vi "driverdata.vi"() -> ()   [LabVIEW 2020]
doc: "This global variable contains data from the FMS system as well as the FRC 4265 Dashboard including safety overrides, calibration commands, and configuration parameters. These data are updated during all robot modes. Robot commands should never be placed in this global variable."
uses:
  <vilib>/Rock Robotics/WPI/DriverStation/WPI_DriverStationRobotMode2.ctl
  <vilib>/Rock Robotics/WPI/DriverStation/WPI_DriverStationAllianceInfo.ctl
panel:
  out "TCP_Override":bool
  out "Starting_TCP_Override":bool
  out "Some_Switch_Armed":bool
  out "Free_Tuning_Variable":dbl
  out "Apply_HUB_Height_Offset":bool
  out "Remaining_Time":dbl
  out "Alliance_Color":T1
  out "Dashboard_Tab":i8
  out "Running_Systems_Check":bool
  out "New_Driver_Profile_Setpoints":dbl[](array[numeric])
  out "Apply_Driver_Profile_Setpoints":bool
  out "Starting_Safety_Override":bool
  out "Starting_IMU_Reset":bool
  out "Field_Oriented_Override":bool
  out "Driver_DPad":T2(ring)
  out "Force_Human_Control":bool
  out "Test_Actuator_Period (s)":dbl
  out "Driver_Joystick_Calibrations":dbl[](array[numeric])
  out "Robot_is_Autonomous":bool
  out "Test_Actuator_Value":dbl
  out "Test_Actuator_Name":string
  out "Disable_Fusion_While_Autonomous":bool
  out "Disable_Fusion_While_Disabled":bool
  out "Camera_Override":bool
  out "Auto_Test_Mode":bool
  out "Clear_Errors":bool
  out "Master_Safety_Override":bool
  out "Auto_Delay (s)":dbl
  out "Home_Wheels":bool
  out "Calibrate_Wheels":bool
  out "Selected_Driver":i32
  out "Selected_Auto_Play":u16
  out "Refresh_Auto_Play_List":bool
  out "Super_Test_Mode":bool
  out "Robot Mode":T3
  # "--FMS--"
  # "--driver joystick--"
  # "--setup and auto--"
  # "--overrides--"
  # "--tune tab--"
  # "--modes--"
  # "--drivebase tuning--"
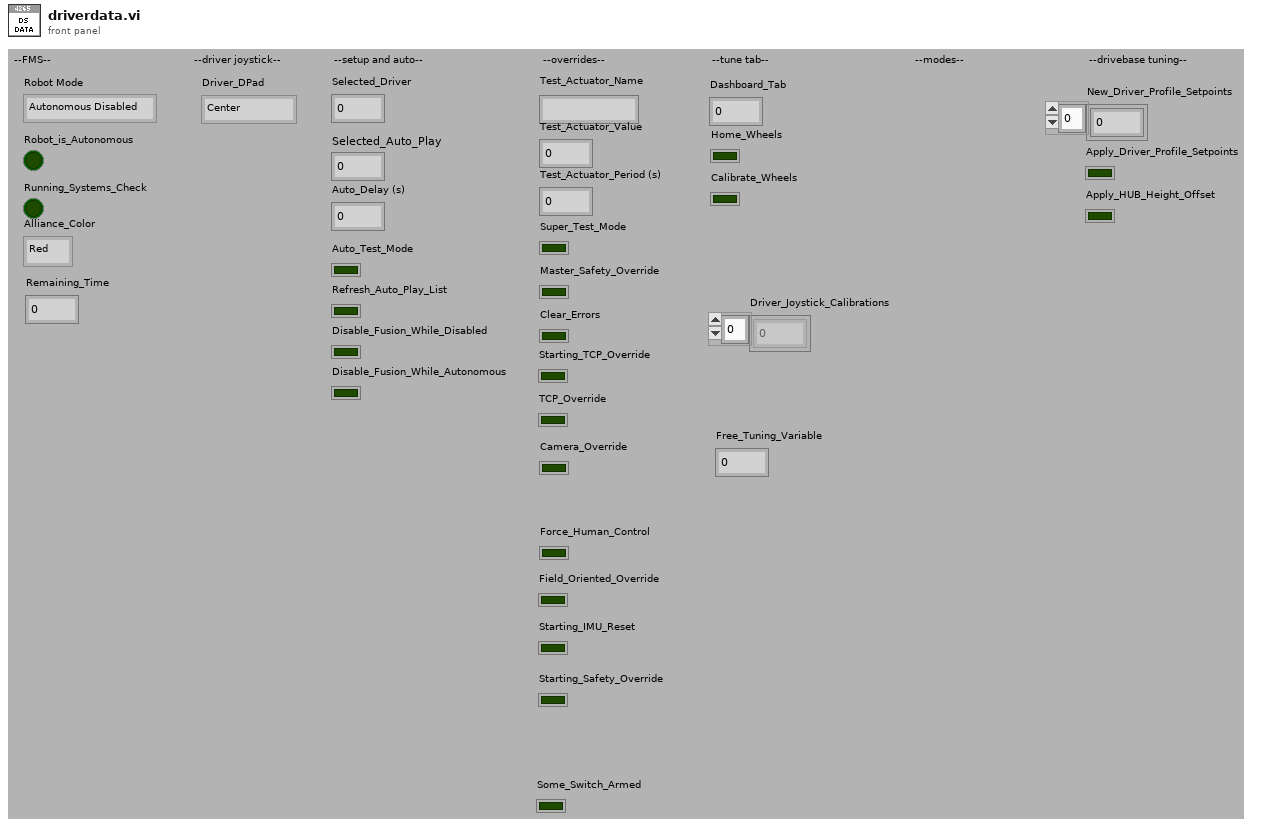
[diagram p1: front panel]
types:
  T1 = typedef "WPI_DriverStationAllianceInfo.ctl" = enum16{"Red", "Blue", "Invalid"}
  T2 = enum16{"Center", "North", "NorthWest", "West", "SouthWest", "South", "SouthEast", "East", "NorthEast"}
  T3 = typedef "WPI_DriverStationRobotMode2.ctl" = enum16{"Autonomous Disabled", "Autonomous Enabled", "Teleop Disabled", "Teleop Enabled", "Disconnected", "Finish", "Test Disabled", "Test Enabled", "Emergency Stopped"}
diagram:
